vi "Send-Receive.vi"(6 "timeout ms (10)":i32=10, 8 "error in (no error)":errorcluster, 9 "bytes to read":i32=12, 10 "request packet":string="\u0000\u0000\u0004\u0000\u0000\u0000ÿÿð8\u0000\u0000\u0000\u0000\u0000\u0001", 11 "TCP Network Connection in":refnum<k5>) -> (0 "error out":errorcluster, 2 "response packet":string, 3 "connection ID out":refnum<k5>)   [LabVIEW 2024, in "OptoMMP.lvlib"]
uses:
  <instrlib>/OptoMMP/OptoMMP.lvlib
panel:
  # "Copyright (c) 2025 California Institute of Technology (Caltech).\nU.S. Government sponsorship acknowledged.\n\nLicensed under the Apache License, Version 2.0 (the \"License\");\nyou may not use this file except in compliance with the License.\nYou may obtain a copy of the License at\n\n    http://www.apache.org/licenses/LICENSE-2.0\n\nUnless required by applicable law or agreed to in writing, software\ndistributed under the License is distributed on an \"AS IS\" BASIS,\nWITHOUT WARRANTIES OR CONDITIONS OF ANY KIND, either express or implied.\nSee the License for the specific language governing permissions and\nlimitations under the License."
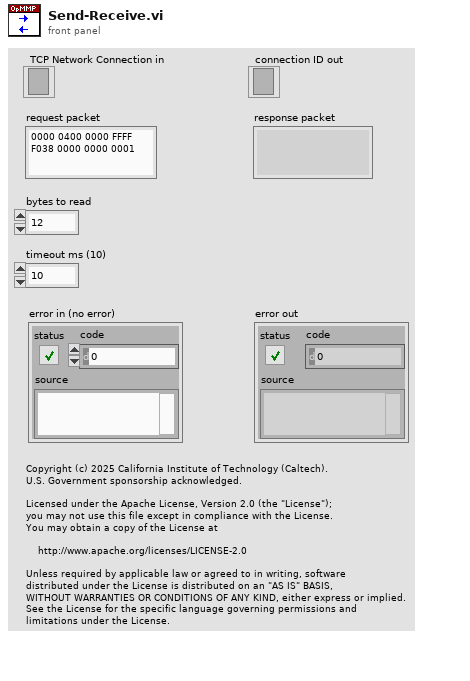
[diagram p1: front panel]
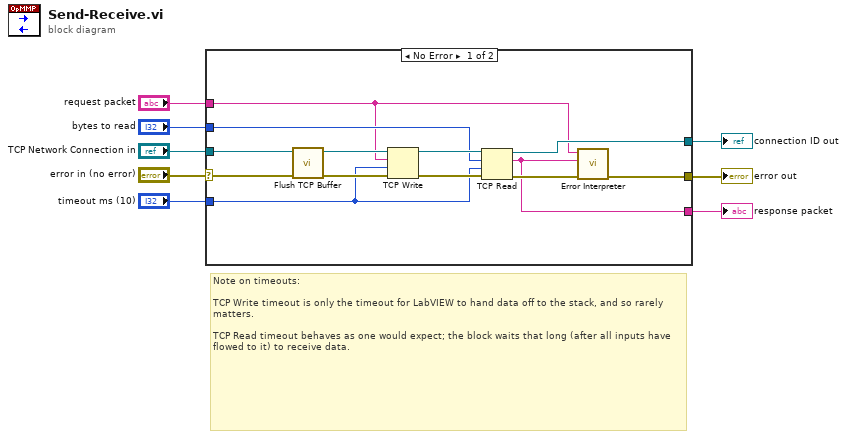
[diagram p0: block diagram]
diagram:
  # "Note on timeouts:\n\nTCP Write timeout is only the timeout for LabVIEW to hand data off to the stack, and so rarely matters.\n\nTCP Read timeout behaves as one would expect; the block waits that long (after all inputs have flowed to it) to receive data."
  n1 = case shown="No Error" "error in (no error)" {
    selector: "error in (no error)" -> [w15 w23]
    tunnel: [w18 w23] -> w8
    tunnel: [w17 w22] -> w7
    tunnel: "TCP Network Connection in" -> [w16 w22]
    tunnel: "request packet" -> [w11 _]
    tunnel: "bytes to read" -> [w12 _]
    tunnel: [w10 _] -> w2
    tunnel: "timeout ms (10)" -> [w9 _]
    frame No Error {
      n2 = call <instrlib>:"Flush TCP Buffer.vi"("error in (no error)"=w15, "TCP Network Connection in"=w16) -> ("error out"=w13:errorcluster, "TCP Network Connection out"=w14:refnum<k5>)  [unwired: 8 in]
      n3 = TCP Write(connection ID=w14, data in=w11, error in (no error)=w13, 9:w9) -> (connection ID out=w20:refnum<k5>, error out=w21:errorcluster)  [unwired: 1 out]
      n4 = TCP Read(connection ID=w20, bytes to read=w12, error in (no error)=w21, 9:w9) -> (connection ID out=w17:refnum<k5>, data out=w10:string, error out=w19:errorcluster)  [unwired: 1 in]
      n5 = call <instrlib>:"Error Interpreter.vi"("request packet"=w11, "response packet"=w10, "error in (no error)"=w19) -> ("error out"=w18:errorcluster)  [unwired: 7 in]
    }
    frame Error {
    }
  }
  "error out" <- w8
  "connection ID out" <- w7
  "response packet" <- w2
